vi "cdaq_anal_adc_process.vi"(8 "error in":errorcluster, 11 "cdaq session":variant) -> (0 "error out":errorcluster)   [LabVIEW 2013]
uses:
  cdaq_anal_session.ctl
  cdaq_anal_adc_command.ctl
  cdaq_anal_adc_data.ctl
  <vilib>/DAQmx/read.llb/DAQmx Read (Analog 1D DBL 1Chan NSamp).vi
  <vilib>/DAQmx/miscellaneous.llb/DAQmx Fill In Error Info.vi
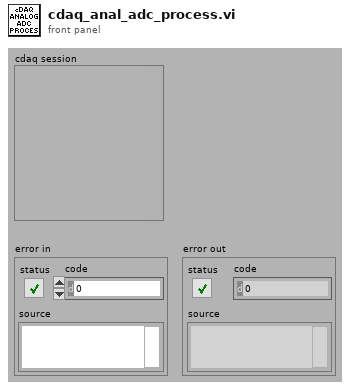
[diagram p1: front panel]
types:
  T1 = typedef "cdaq_anal_session.ctl" = cluster{"mclk [Hz]":dbl, "DAC device":tag, "ADC device":tag, "DAC task":refnum<k21>, "ADC task":refnum<k21>, "adc idn":string, "dac idn":string, "fs [Hz]":dbl, "queue adc cmd":refnum<queue>, "queue adc data":refnum<queue>, "adc proc ref":refnum<vi>}
  T2 = typedef "cdaq_anal_adc_data.ctl" = cluster{"wave":dbl[], "timestamp [s]":dbl}
  T3 = typedef "cdaq_anal_adc_command.ctl" = cluster{"sample to get":i32, "stop":bool}
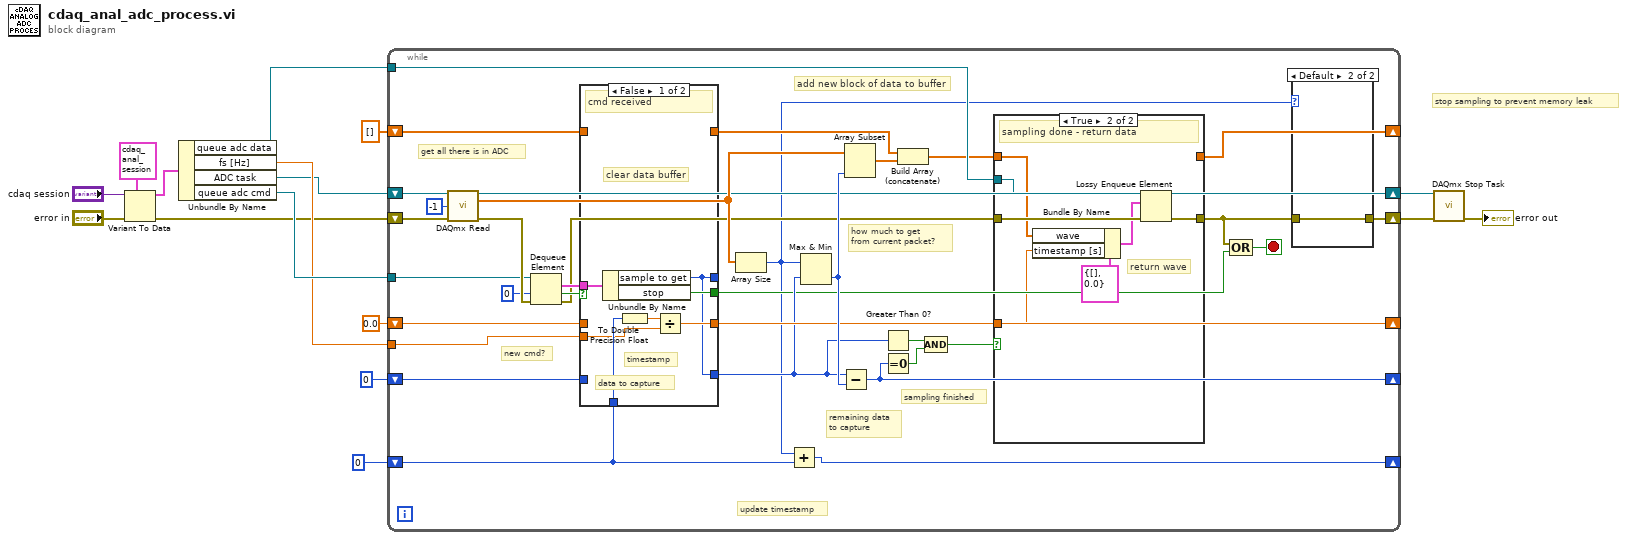
[diagram p0: block diagram]
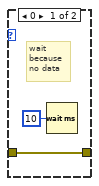
[diagram p2: hidden frame]
diagram:
  # "stop sampling to prevent memory leak"
  n1 = Variant To Data(error in="error in", type=T1 {"mclk [Hz]"=0.0, "DAC device"="", "ADC device"="", "DAC task"="", "ADC task"="", "adc idn"="", "dac idn"="", "fs [Hz]"=0.0, "queue adc cmd"=refnum, "queue adc data"=refnum, "adc proc ref"=refnum} ("cdaq session"), Variant="cdaq session") -> (data=w13:T1, error out=w2:errorcluster)
  n2 = Unbundle By Name(w13) -> ("queue adc data"=w7:refnum<queue>, "fs [Hz]"=w8:dbl, "ADC task"=w1:refnum<k21>, "queue adc cmd"=w12:refnum<queue>)
  n3 = while {
    shift-right: [w20] -> w5
    shift-left: w2 -> [w50]
    shift-right: [w31] -> w3
    shift-left: w1 -> [w49]
    shift-right: [w37] -> _
    shift-left: i64 0 -> [w39]
    tunnel: w12 -> [w46]
    shift-right: [w34] -> _
    shift-left: 0 -> [w25]
    shift-right: [w23] -> _
    shift-left: dbl[] [] -> [w36]
    shift-right: [w27] -> _
    shift-left: 0.0 -> [w17]
    tunnel: w8 -> [w38]
    tunnel: w7 -> [w28]
    stop <- w21 stop-if-true
    # "new cmd?"
    # "get all there is in ADC"
    # "sampling finished"
    # "update timestamp"
    # "add new block of data to buffer"
    # "remaining data\nto capture"
    # "how much to get\nfrom current packet?"
    n4 = call-poly <vilib>:"DAQmx Read.vi"("task/channels in"=w49, "number of samples per channel"=-1, "error in"=w50) -> ("task out"=w31:refnum<k21>, "data"=w42:dbl[], "error out"=w47:errorcluster)  [unwired: 10 in]
    n5 = Dequeue Element(queue=w46, timeout in ms (-1)=0, error in (no error)=w47) -> (element=w44:T3, timed out?=w43:bool, error out=w29:errorcluster)  [unwired: 1 out]
    n6 = case shown="False" w43 {
      tunnel: w44 -> [w69 _]
      tunnel: [w68 _] -> w22
      tunnel: [w63 _] -> _
      tunnel: w39 -> [w67 _]
      tunnel: w38 -> [w65 _]
      tunnel: [w64 w70] -> w27
      tunnel: [_ w72] -> w35
      tunnel: w36 -> [_ w72]
      tunnel: [w63 w71] -> w24
      tunnel: w25 -> [_ w71]
      tunnel: w17 -> [_ w70]
      frame False {
        # "data to capture"
        # "clear data buffer"
        # "timestamp"
        # "cmd received"
        n7 = Unbundle By Name(w69) -> ("sample to get"=w63:i32, "stop"=w68:bool)
        n8 = To Double Precision Float(number=w67) -> (double precision float=w66:dbl)
        n9 = Divide(x=w66, y=w65) -> (x/y=w64:dbl)
      }
      frame True {
        # "timeout"
      }
    }
    n10 = Array Size(array=w42) -> (size(s)=w18:i32)
    n11 = Add(x=w18, y=w39) -> (x+y=w37:i64)
    n12 = Max & Min(x=w18, y=w24) -> (min(x,y)=w41:i32)  [unwired: 1 out]
    n13 = Subtract(x=w24, y=w41) -> (x-y=w34:i32)
    n14 = Array Subset(array=w42, length=w41) -> (w40:dbl[])  [unwired: 1 in]
    n15 = Greater Than 0?(x=w24) -> (x > 0?=w33:bool)
    n16 = Equal To 0?(x=w34) -> (x = 0?=w32:bool)
    n17 = Build Array (concatenate)(w35, w40) -> (w26:dbl[])
    n18 = Compound Arithmetic op=AND(w33, w32) -> (w30:bool)
    n19 = case shown="True" w30 {
      tunnel: w29 -> [w54 w62]
      tunnel: w28 -> [_ w61]
      tunnel: w27 -> [_ w59]
      tunnel: w26 -> [w55 w57]
      tunnel: [w55 _] -> w23
      tunnel: [w54 w56] -> w19
      frame False {
      }
      frame True {
        # "return wave"
        # "sampling done - return data"
        n20 = Bundle By Name(cluster=T2 {"wave"=[], "timestamp [s]"=0.0} ("adc data"), "wave"=w57, "timestamp [s]"=w59) -> (w58:T2)
        n21 = Lossy Enqueue Element(queue=w61, element=w58, error in (no error)=w62) -> (error out=w56:errorcluster)  [unwired: 3 out]
      }
    }
    n22 = Compound Arithmetic op=OR(w19, w22) -> (w21:bool)
    n23 = case shown="Default" w18 {
      tunnel: [w52 w53] -> w20
      tunnel: w19 -> [w52 w53]
      frame 0 {
        # "wait\nbecause\nno data"
        n24 = Wait (ms)(milliseconds to wait=u32 10) -> ()  [unwired: 1 out]
      }
      frame Default {
      }
    }
  }
  n25 = call <vilib>:"DAQmx Stop Task.vi"("task/channels in"=w3, "error in"=w5) -> ("error out"=→"error out":errorcluster)  [unwired: 12 in, 1 out]
